vi "Close Debug File.vi"(4 "error in (no error)":errorcluster, 7 "Debug refnum":T1) -> (0 "error out":errorcluster)   [LabVIEW 2011]
uses:
  <vilib>/Utility/config.llb/Config Data RefNum.ctl
  <vilib>/Utility/config.llb/NI_LVConfig.lvlib
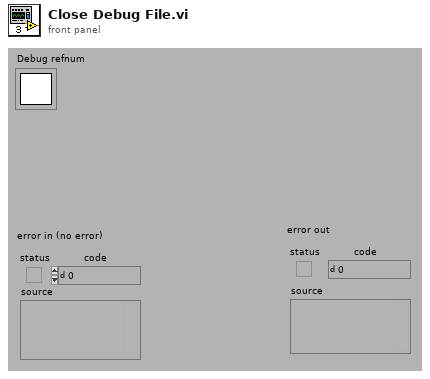
[diagram p1: front panel]
types:
  T1 = typedef "NI_LVConfig.lvlib/Config Data RefNum.ctl" = refnum<k1>
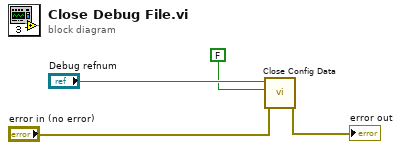
[diagram p0: block diagram]
diagram:
  n1 = call <vilib>:"Close Config Data.vi"("error in (no error)"="error in (no error)", "write file if changed (T)"=FALSE, "refnum"="Debug refnum") -> ("error out"=→"error out":errorcluster)  [unwired: 8 out]
